vi "Delete Node.vi"(6 "Remove Children? (T)":bool=TRUE, 8 "error in (no error)":errorcluster, 10 "UID":string, 11 "Base Tree in":refnum<class "Base Tree.lvclass">) -> (0 "error out":errorcluster, 3 "Base Tree out":refnum<class "Base Tree.lvclass">)   [LabVIEW 2017, in "opcua.lvlib" / "Browser Core.lvlib" / "Base Tree.lvclass"]
doc: "Remove Node with given UID from the Tree. By default, removing the given node will also remove all children recursively."
uses:
  Base Tree.lvclass
  Base Tree.lvclass/Base Tree.ctl
  Node Classes/Generic Node/Generic Node.lvclass
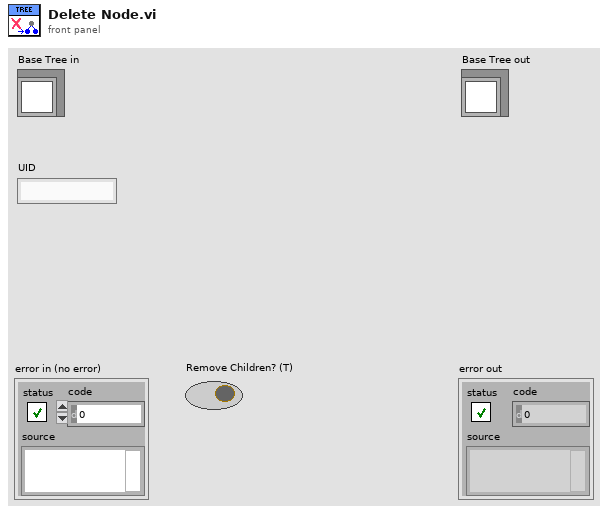
[diagram p1: front panel]
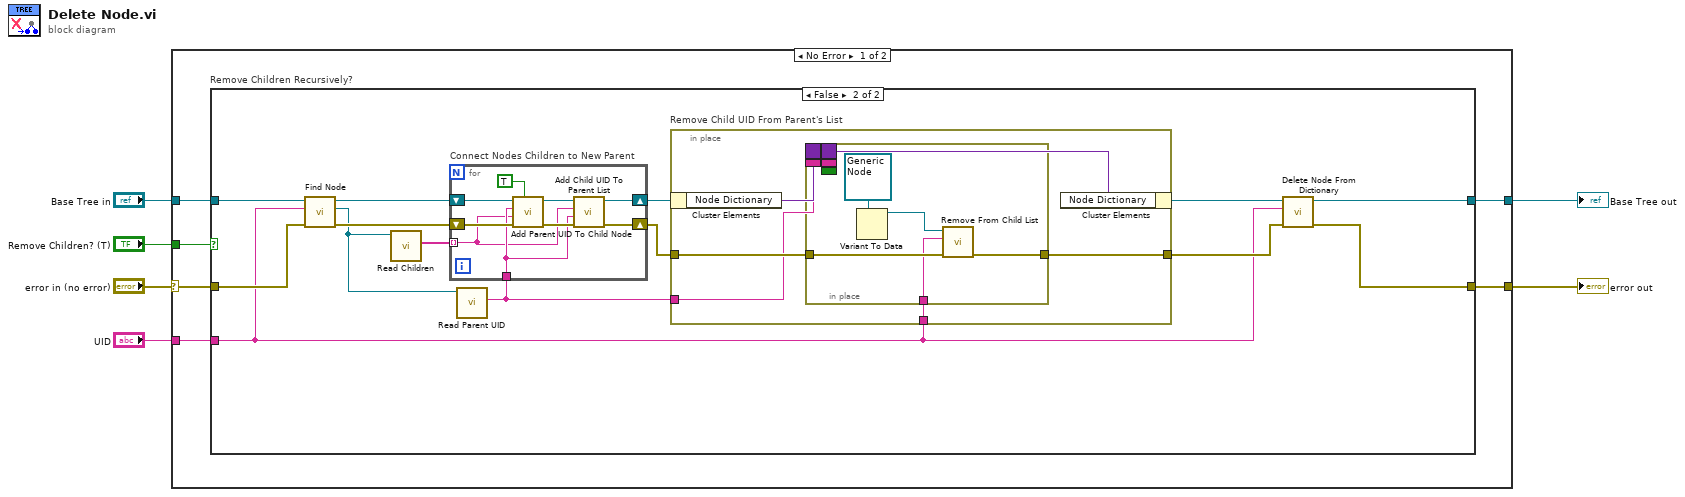
[diagram p0: block diagram]
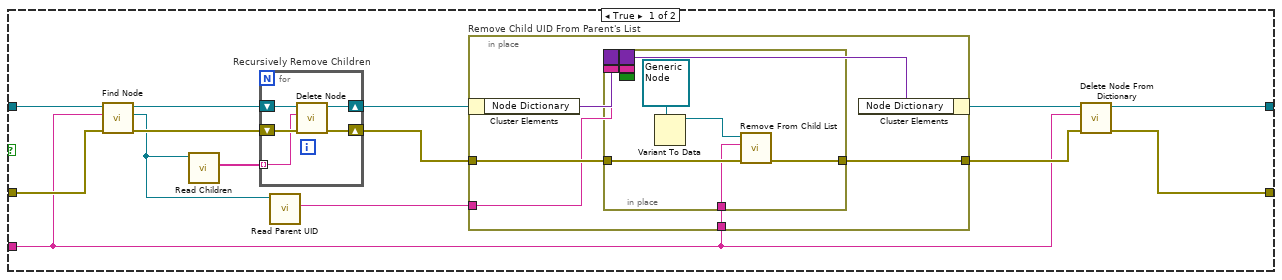
[diagram p2: hidden frame]
diagram:
  n1 = case shown="No Error" "error in (no error)" {
    selector: "error in (no error)" -> [w9 w82]
    tunnel: [w8 w82] -> w5
    tunnel: [w7 w81] -> w3
    tunnel: "Base Tree in" -> [w10 w81]
    tunnel: "UID" -> [w11 _]
    tunnel: "Remove Children? (T)" -> [w12 _]
    frame No Error {
      n2 = case "Remove Children Recursively?" shown="False" w12 {
        tunnel: w11 -> [w17 w46]
        tunnel: w10 -> [w26 w58]
        tunnel: w9 -> [w24 w56]
        tunnel: [w16 w49] -> w8
        tunnel: [w15 w48] -> w7
        frame True {
          n3 = call-dynamic "Find Node.vi"("error in (no error)"=w24, "UID"=w17, "Base Tree in"=w26) -> ("error out"=w23:errorcluster, "Node"=w21:refnum<class "Generic Node.lvclass">, "Base Tree out"=w25:refnum<class "Base Tree.lvclass">)  [unwired: 5 in, 1 out]
          n4 = call "Read Children.vi"("Generic Node in"=w21) -> ("Children"=w22:string[])  [unwired: 8 in, 2 out]
          n5 = for "Recursively Remove Children" {
            shift-right: [w41] -> w19
            shift-left: w23 -> [w43]
            tunnel: w22 -> [w42] mode=indexing
            shift-right: [w40] -> w20
            shift-left: w25 -> [w44]
            n6 = call-dynamic "Delete Node.vi"("error in (no error)"=w43, "UID"=w42, "Base Tree in"=w44) -> ("error out"=w41:errorcluster, "Base Tree out"=w40:refnum<class "Base Tree.lvclass">)  [unwired: 7 in]
          }
          n7 = call "Read Parent UID.vi"("Generic Node in"=w21) -> ("Parent UID"=w14:string)  [unwired: 8 in, 2 out]
          n8 = in-place "Remove Child UID From Parent's List" {
            in-place-border: w19 -> [w32]
            in-place-border: [w31] -> w18
            in-place-border: w17 -> [w30]
            in-place-border: w14 -> [w28]
            n9 = in-place-cluster #1(w20) -> ("Node Dictionary"=w29:variant)
            n10 = in-place {
              in-place-border: w32 -> [w39]
              in-place-border: [w38] -> w31
              in-place-border: w30 -> [w37]
              border: w29 -> [_]
              border: w28 -> [_]
              border: [_] -> w27
              border: _ -> [_]
              border: _ -> [_]
              n11 = Variant To Data(type=refnum<class "Generic Node.lvclass"> refnum ("Browser Core.lvlib:Generic Node.lvclass"), Variant=w36) -> (data=w34:refnum<class "Generic Node.lvclass">)  [unwired: 1 in, 1 out]
              n12 = call "Remove From Child List.vi"("error in (no error)"=w39, "Child ID"=w37, "Generic Node in"=w34) -> ("error out"=w38:errorcluster, "Generic Node out"=w33:refnum<class "Generic Node.lvclass">)  [unwired: 7 in]
            }
            n13 = in-place-cluster #1("Node Dictionary"=w27) -> (w13:refnum<class "Base Tree.lvclass">)
          }
          n14 = call "Delete Node From Dictionary.vi"("error in (no error)"=w18, "UID"=w17, "Base Tree in"=w13) -> ("error out"=w16:errorcluster, "Base Tree out"=w15:refnum<class "Base Tree.lvclass">)  [unwired: 7 in]
        }
        frame False {
          n15 = call-dynamic "Find Node.vi"("error in (no error)"=w56, "UID"=w46, "Base Tree in"=w58) -> ("error out"=w55:errorcluster, "Node"=w53:refnum<class "Generic Node.lvclass">, "Base Tree out"=w57:refnum<class "Base Tree.lvclass">)  [unwired: 5 in, 1 out]
          n16 = call "Read Children.vi"("Generic Node in"=w53) -> ("Children"=w54:string[])  [unwired: 8 in, 2 out]
          n17 = call "Read Parent UID.vi"("Generic Node in"=w53) -> ("Parent UID"=w45:string)  [unwired: 8 in, 2 out]
          n18 = for "Connect Nodes Children to New Parent" {
            shift-right: [w75] -> w51
            shift-left: w55 -> [w79]
            tunnel: w54 -> [w72] mode=indexing
            shift-right: [w76] -> w52
            shift-left: w57 -> [w80]
            tunnel: w45 -> [w73]
            n19 = call "Add Parent UID To Child Node.vi"("Replace? (F)"=TRUE, "error in (no error)"=w79, "Child UID"=w72, "Parent UID"=w73, "Base Tree in"=w80) -> ("error out"=w74:errorcluster, "Base Tree out"=w77:refnum<class "Base Tree.lvclass">)  [unwired: 4 in, 1 out]
            n20 = call "Add Child UID To Parent List.vi"("Base Tree in"=w77, "UID"=w72, "ParentUID"=w73, "error in (no error)"=w74) -> ("Base Tree out"=w76:refnum<class "Base Tree.lvclass">, "error out"=w75:errorcluster)  [unwired: 5 in]
          }
          n21 = in-place "Remove Child UID From Parent's List" {
            in-place-border: w51 -> [w64]
            in-place-border: [w63] -> w50
            in-place-border: w46 -> [w62]
            in-place-border: w45 -> [w60]
            n22 = in-place-cluster #2(w52) -> ("Node Dictionary"=w61:variant)
            n23 = in-place {
              in-place-border: w64 -> [w71]
              in-place-border: [w70] -> w63
              in-place-border: w62 -> [w69]
              border: w61 -> [_]
              border: w60 -> [_]
              border: [_] -> w59
              border: _ -> [_]
              border: _ -> [_]
              n24 = Variant To Data(type=refnum<class "Generic Node.lvclass"> refnum ("Browser Core.lvlib:Generic Node.lvclass"), Variant=w68) -> (data=w66:refnum<class "Generic Node.lvclass">)  [unwired: 1 in, 1 out]
              n25 = call "Remove From Child List.vi"("error in (no error)"=w71, "Child ID"=w69, "Generic Node in"=w66) -> ("error out"=w70:errorcluster, "Generic Node out"=w65:refnum<class "Generic Node.lvclass">)  [unwired: 7 in]
            }
            n26 = in-place-cluster #2("Node Dictionary"=w59) -> (w47:refnum<class "Base Tree.lvclass">)
          }
          n27 = call "Delete Node From Dictionary.vi"("error in (no error)"=w50, "UID"=w46, "Base Tree in"=w47) -> ("error out"=w49:errorcluster, "Base Tree out"=w48:refnum<class "Base Tree.lvclass">)  [unwired: 7 in]
        }
      }
    }
    frame Error {
      # "Do Not Edit Tree on Error In"
    }
  }
  "error out" <- w5
  "Base Tree out" <- w3
